vi "Teleop.vi"(10 "Match Info":T4={"Autonomous Elapsed Seconds"=0.0, "TeleOp Elapsed Seconds"=0.0, "Disabled Elapsed Seconds"=0.0, "Visited Autonomous"=FALSE, "Visited TeleOp"=FALSE, "Visited Disabled"=FALSE, "Autonomous Settings"={"Autonomous Style"=enum."Independent", "VI Refnum"=refnum}}, 11 "Call Context":T5) -> ()   [LabVIEW 2013]
doc: "This VI is called for each TeleOp packet received from the DS where the robot is not disabled. It is often used to read from the joysticks and update I/O or to update setpoints for timed control loops. It should complete and return within 20 milliseconds or it may miss DS packets."
uses:
  <vilib>/Rock Robotics/WPI/DriverStation/WPI_DriverStationDerivedRobotMode.ctl
  <vilib>/Rock Robotics/WPI/DriverStation/WPI_DriverStationMatch Info.ctl
  <vilib>/Rock Robotics/WPI/Solenoid/WPI_SolenoidValue.ctl
  <vilib>/Rock Robotics/WPI/Relay/WPI_RelayValue.ctl
  Robot Global Data.vi
  <vilib>/Rock Robotics/Network Tables/SD Read Number.vi
  <vilib>/Rock Robotics/WPI/Solenoid/WPI_SolenoidGetEnum.vi
  <vilib>/Rock Robotics/WPI/Solenoid/WPI_SolenoidSetEnum.vi
  <vilib>/Rock Robotics/WPI/Compressor/WPI_CompressorGetSetRefNum.vi
  <vilib>/Rock Robotics/WPI/Joystick/WPI_JoystickGetSetRefNum.vi
  <vilib>/Rock Robotics/WPI/RobotDrive/WPI_RobotDriveGetSetRefNum.vi
panel:
  out "Waveform Chart 4":dbl(graph)
  out "Waveform Chart 3":dbl(graph)
  in  "Grabber Timer":dbl
  in  "GrabberCurrentTarget":dbl
  in  "HasGrabberBeenReset":bool
  in  "ToughBoxEncoderTopPosition":dbl
  in  "Current Grabber Status":T1(ring)
  out "Waveform Chart 2":dbl(graph)
  in  "Run Grabber PID 2":bool
  out "Reed Switch 2":bool
  out "Reed Switch 1":bool
  out "Top Limit Tripped":bool
  out "Micro Switch":bool
  out "Bottom Limit Tripped":bool
  out "Axis Value  6":dbl
  out "Axis Value 5":dbl
  out "Axis Value 4":dbl
  in  "Grabber Axis Value":T2(ring)
  in  "Current Shooter Status":T3(ring)
  out "Waveform Chart":dbl(graph)
  out "Mechanism Moving Up":bool
  out "Mechanism Moving Down":bool
  out "Time Since Button Pressed":dbl
  in  "Manual Override Activated":bool
  in  "Button 2 Pressed":bool
  in  "Firing Pin Forward":bool
  in  "Mechanism Piston Forward":bool
  in  "Tick Taken":bool
  out "Time at Gather":dbl
  out "Timer for firing mech":dbl
  in  "Mechanism Status":string
types:
  T1 = enum16{"Resetting", "Going Up", "Going Up Slow", "In Shooting Position", "Going Down", "Going Down Slow", "In Loading Position"}
  T2 = enum16{"Less Than Zero", "Greater Than Zero", "Equal To Zero"}
  T3 = enum16{"Retracting", "Firing", "Ready to fire", "Pulling back", "Just fired"}
  T4 = typedef "WPI_DriverStationMatch Info.ctl" = cluster{"Autonomous Elapsed Seconds":dbl, "TeleOp Elapsed Seconds":dbl, "Disabled Elapsed Seconds":dbl, "Visited Autonomous":bool, "Visited TeleOp":bool, "Visited Disabled":bool, "Autonomous Settings":cluster{"Autonomous Style":enum16{"Iterative", "Independent"}, "VI Refnum":refnum<vi>}}
  T5 = typedef "WPI_DriverStationDerivedRobotMode.ctl" = enum16{"Init", "Execute", "Stop"}
  T6 = typedef "WPI_SolenoidValue.ctl" = enum16{"Off", "On", "Forward", "Reverse"}
  T7 = enum16{"Resetting", "Going Up", "Going Up Slow", "In Shooting Position", "Going Down", "Going Down Slow", "In Loading Position", ""}
  T8 = typedef "WPI_MotorControlDeviceRef.ctl" = cluster{"DeviceStatus":errorcluster, "Type":enum16{"PWM", "CAN"}, "PWM":cluster{"Digital Module":T9, "PWM Channel":T10, "DeadBand":T11}, "CAN":cluster{"Device Number":u8, "Control Mode":T12, "Semaphore":T13, "Max Vout":dbl}, "Invert":bool, "TransformRef":T14, "InvTransformRef":T14}
  T9 = typedef "FPGA_TypedefDigitalModule.ctl" = enum16{"Digital Module 1", "Digital Module 2"}
  T10 = typedef "FPGA_DIOPWMChannel.ctl" = enum8{"PWM 1", "PWM 2", "PWM 3", "PWM 4", "PWM 5", "PWM 6", "PWM 7", "PWM 8", "PWM 9", "PWM 10", "Invalid"}
  T11 = typedef "WPI_PWMDeadband.ctl" = cluster{"Name":string, "maxPositivePwm":i32, "minPositivePwm":i32, "centerPwm":i32, "maxNegativePwm":i32, "minNegativePwm":i32, "angularRange":u16}
  T12 = typedef "WPI_CANJaguar_ControlMode.ctl" = enum8{"Percent VBus", "Current", "Speed", "Position", "Voltage"}
  T13 = typedef "Semaphore RefNum" = refnum<k1>
  T14 = typedef "WPI_PWMTransform_ConPane.ctl" = refnum<vi>
  T15 = typedef "WPI_SolenoidDevRef.ctl" = cluster{"DevStatus":errorcluster, "Solenoid Module":T16, "Forward Solenoid Channel":T17, "Reverse Solenoid Channel":T17}
  T16 = typedef "FPGA_TypedefSolenoidModule.ctl" = enum16{"Solenoid Module 1", "Solenoid Module 2"}
  T17 = typedef "WPI_SolenoidChannel.ctl" = enum8{"Solenoid 1", "Solenoid 2", "Solenoid 3", "Solenoid 4", "Solenoid 5", "Solenoid 6", "Solenoid 7", "Solenoid 8", "Invalid"}
  T18 = typedef "WPI_JoystickDevRef.ctl" = cluster{"Device":T19}
  T19 = typedef "WPI_JoystickDeviceEnum.ctl" = enum16{"USB 1", "USB 2", "USB 3", "USB 4", "Kinect 1", "Kinect 2"}
  T20 = typedef "WPI_JoystickButtonState.ctl" = cluster{"Button 1":bool, "Button 2":bool, "Button 3":bool, "Button 4":bool, "Button 5":bool, "Button 6":bool, "Button 7":bool, "Button 8":bool, "Button 9":bool, "Button 10":bool, "Button 11":bool, "Button 12":bool}
  T21 = typedef "WPI_DigitalInputDevRef.ctl" = cluster{"DevStatus":errorcluster, "DIO Channel":T22, "Digital Module":T9}
  T22 = typedef "FPGA_DIOChannel.ctl" = enum8{"DIO 1", "DIO 2", "DIO 3", "DIO 4", "DIO 5", "DIO 6", "DIO 7", "DIO 8", "DIO 9", "DIO 10", "DIO 11", "DIO 12", "DIO 13", "DIO 14", "Invalid"}
  T23 = typedef "WPI_EncoderDevRef.ctl" = cluster{"DevStatus":errorcluster, "EncoderIndex":T24, "CounterIndex":T25, "DistancePerCount":dbl, "Decoding Type":T26}
  T24 = typedef "FPGA_EncoderIdx.ctl" = enum8{"Enc 0", "Enc 1", "Enc 2", "Enc 3", "Invalid"}
  T25 = typedef "FPGA_CounterCtrSystemIndex.ctl" = enum8{"Ctr 0", "Ctr 1", "Ctr 2", "Ctr 3", "Ctr 4", "Ctr 5", "Ctr 6", "Ctr 7", "Invalid"}
  T26 = typedef "WPI_EncoderType.ctl" = enum16{"1x", "2x", "4x"}
  T27 = typedef "WPI_RelayDevRef.ctl" = cluster{"DevStatus":errorcluster, "Relay Channel":T28, "Digital Module":T9, "Relay Direction":T29}
  T28 = typedef "FPGA_DIORelayChannel.ctl" = enum8{"Relay 1", "Relay 2", "Relay 3", "Relay 4", "Relay 5", "Relay 6", "Relay 7", "Relay 8", "Invalid"}
  T29 = typedef "WPI_RelayDirection.ctl" = enum16{"Both directions", "Forward only", "Reverse only"}
  T30 = typedef "WPI_CompressorDevRef.ctl" = cluster{"DevStatus":errorcluster, "DigitalInputDevRef":T21, "RelayDevRef":T27}
  T31 = typedef "WPI_RelayValue.ctl" = enum16{"Off", "On", "Forward", "Reverse"}
  T32 = typedef "WPI_AnalogChannelDevRef.ctl" = cluster{"DevStatus":errorcluster, "Analog Module":T33, "Analog Channel":T34}
  T33 = typedef "FPGA_TypedefAnalogModule.ctl" = enum16{"Analog Module 1", "Analog Module 2"}
  T34 = typedef "FPGA_AIChannel.ctl" = enum8{"AI 1", "AI 2", "AI 3", "AI 4", "AI 5", "AI 6", "AI 7", "AI 8", "Invalid"}
  T35 = typedef "WPI_ServoDeviceRef.ctl" = cluster{"DeviceStatus":errorcluster, "Digital Module":T9, "PWM Channel":T10, "DeadBand":T11}
  T36 = cluster{"axis 1 (x)":dbl, "axis 2 (y)":dbl, "axis 3 (throttle)":dbl, "axis 4":dbl, "axis 5":dbl, "axis 6":dbl}
  T37 = typedef "WPI_RobotDriveDevRef.ctl" = cluster{"DevStatus":errorcluster, "Motors[]":T8[], "Square Inputs":bool, "Max Output":dbl, "Isochronous":bool}
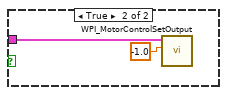
[diagram p2: hidden frame]
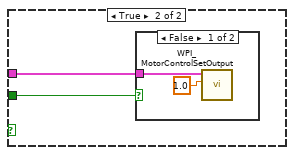
[diagram p3: hidden frame]
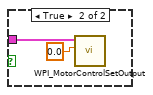
[diagram p4: hidden frame]
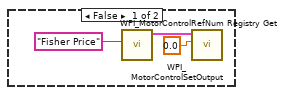
[diagram p5: hidden frame]
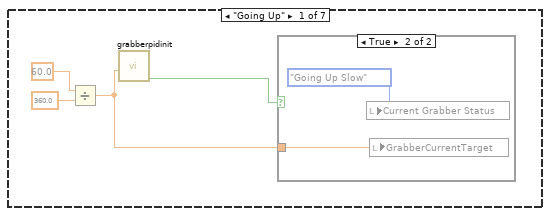
[diagram p7: hidden frame]
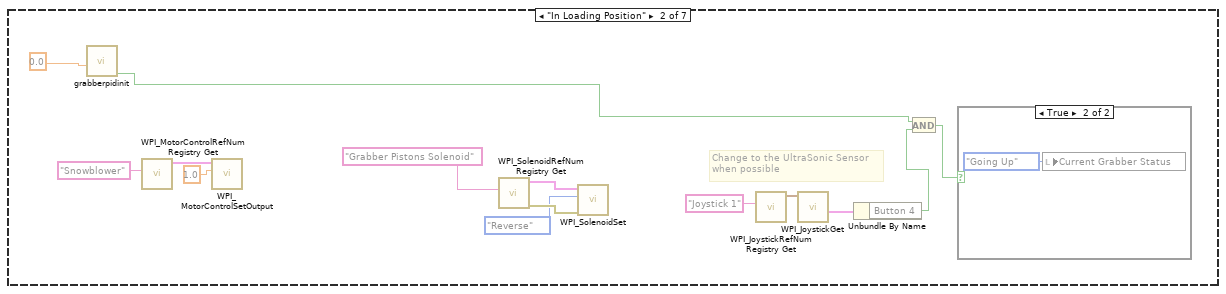
[diagram p9: hidden frame]
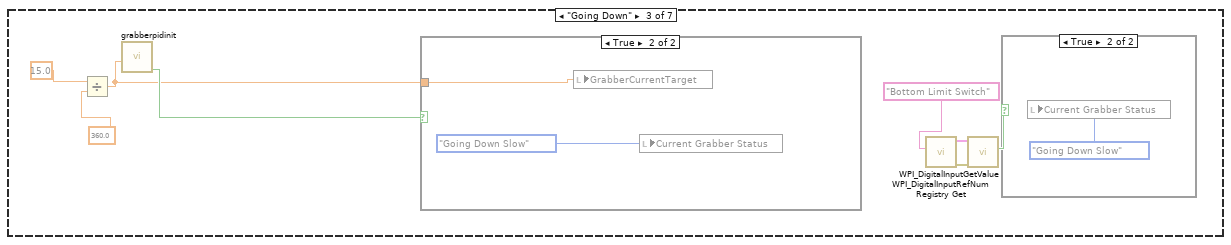
[diagram p11: hidden frame]
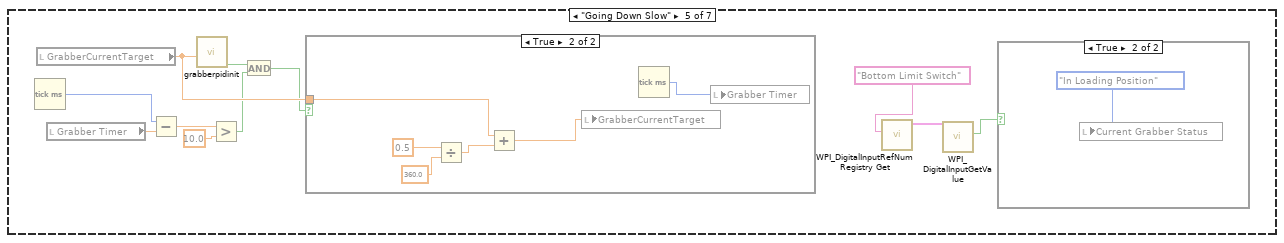
[diagram p15: hidden frame]
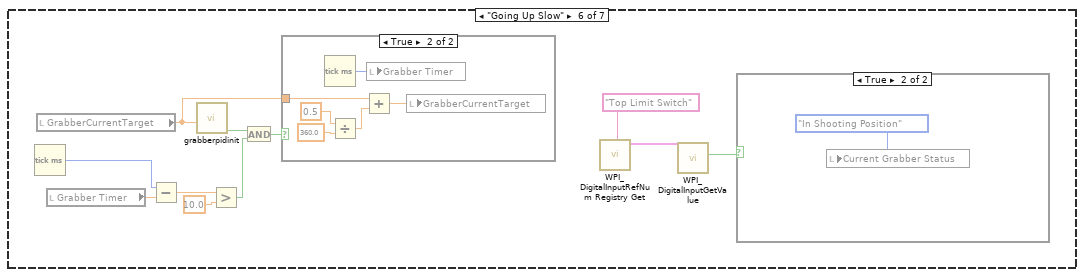
[diagram p18: hidden frame]
diagram:
  (unwired) "Below code is for running the Raising/Lowering motors"
  (unwired) "This code sets the toggle rate used by the Periodic Tasks VI.  For teleop mode we flash the USER1 LED on the cRIO at a fast rate.  Look at the Periodic Tasks VI to see how this global value is used."
  (unwired) "This VI is called each time a TeleOp DS packet is received.  Use it to respond to new joystick or Driver Station values.\n\nCommon tasks include reading the joysticks and updating motors, and updating setpoints for periodic loops.\n\nYou can open I/O on the FIRST Call, or in the Begin.vi."
  # "Top Limit Switch may need invert"
  # "one encoder"
  # "Check me!"
  # "If no buttons pressed - 0\nIf left pressed = 7\nIf right pressed = -7\nIf both = 0"
  # "Publish the Robot Drive Motor\nvalues to the dashboard"
  # "Publish the joystick data the\nrobot sees to the dashboard"
  # "Each time we enter, report that\nwe are running teleop"
  # "Use to differentiate between\nFirst, Last, and Intermediate calls"
  # "Read Joystick X and Y values and update motor values"
  n1 = call <vilib>:"SD Read Boolean.vi"("Name"="Manual Mechanism Override") -> ("Boolean"=w54:bool)  [unwired: 8 in, 2 out]
  n2 = disable-structure shown="Disabled" {
    disable-tunnel: w54 -> [w153 _]
    frame Disabled {
      n3 = Not(x=w153) -> (.not. x?=w154:bool)
      n4 = case shown="True" w154 {
        frame False {
        }
        frame True {
          n5 = local read "Current Grabber Status"() -> (w155:T1)
          n6 = case shown="\"In Shooting Position\"" w155 {
            frame "Going Up" {
              n7 = Divide(x=60.0 ("setpoint"), y=360.0) -> (x/y=w158:dbl)
              n8 = call "grabberpidinit.vi"("setpoint"=w158) -> ("Done? 2"=w159:bool)  [unwired: 10 in]
              n9 = case shown="True" w159 {
                tunnel: w158 -> [_ w160]
                frame False {
                }
                frame True {
                  n10 = local write "Current Grabber Status"(T1."Going Up Slow" ("Current Grabber Status")) -> ()
                  n11 = local write "GrabberCurrentTarget"(w160) -> ()
                }
              }
            }
            frame "In Loading Position" {
              # "Change to the UltraSonic Sensor\nwhen possible"
              n12 = call "grabberpidinit.vi"("setpoint"=0.0) -> ("Done? 2"=w162:bool)  [unwired: 10 in]
              n13 = call <vilib>:"WPI_MotorControlRefNum Registry Get.vi"("refnum name"="Snowblower") -> ("MotorControlDevRef"=w174:T8)  [unwired: 9 in, 1 out]
              n14 = call <vilib>:"WPI_MotorControlSetOutput.vi"("Output"=1.0, "MotorControlDevRef"=w174) -> ()  [unwired: 7 in, 3 out]
              n15 = call <vilib>:"WPI_SolenoidRefNum Registry Get.vi"("refnum name"="Grabber Pistons Solenoid") -> ("error out"=w171:errorcluster, "SolenoidDevRef"=w170:T15)  [unwired: 9 in]
              n16 = call-poly <vilib>:"WPI_SolenoidSet.vi"("error in (no error)"=w171, "Value"=WPI_SolenoidValue."Reverse", "SolenoidDevRef"=w170) -> ()  [unwired: 7 in, 2 out]
              n17 = call <vilib>:"WPI_JoystickRefNum Registry Get.vi"("refnum name"="Joystick 1") -> ("JoystickDevRef"=w166:T18)  [unwired: 1 in, 9 out]
              n18 = call <vilib>:"WPI_JoystickGet.vi"("JoystickDevRef"=w166) -> ("Buttons"=w165:T20)  [unwired: 1 in, 5 out]
              n19 = Unbundle By Name(w165) -> ("Button 4"=w163:bool)
              n20 = And(x=w162, y=w163) -> (x .and. y?=w164:bool)
              n21 = case shown="True" w164 {
                frame False {
                }
                frame True {
                  n22 = local write "Current Grabber Status"(T1."Going Up" ("Current Grabber Status")) -> ()
                }
              }
            }
            frame "Going Down" {
              n23 = Divide(x=15.0, y=360.0) -> (x/y=w181:dbl)
              n24 = call "grabberpidinit.vi"("setpoint"=w181) -> ("Done? 2"=w182:bool)  [unwired: 10 in]
              n25 = case shown="True" w182 {
                tunnel: w181 -> [_ w187]
                frame False {
                }
                frame True {
                  n26 = local write "GrabberCurrentTarget"(w187) -> ()
                  n27 = local write "Current Grabber Status"(T1."Going Down Slow" ("Current Grabber Status")) -> ()
                }
              }
              n28 = call <vilib>:"WPI_DigitalInputRefNum Registry Get.vi"("refnum name"="Bottom Limit Switch") -> ("error out"=w179:errorcluster, "DigitalInputDevRef"=w178:T21)  [unwired: 9 in]
              n29 = call <vilib>:"WPI_DigitalInputGetValue.vi"("error in (no error)"=w179, "DigitalInputDevRef"=w178) -> ("Value"=w177:bool)  [unwired: 7 in, 2 out]
              n30 = case shown="True" w177 {
                frame False {
                }
                frame True {
                  n31 = local write "Current Grabber Status"(T1."Going Down Slow" ("Current Grabber Status")) -> ()
                }
              }
            }
            frame "In Shooting Position" {
              n32 = local read "ToughBoxEncoderTopPosition"() -> (w189:dbl)
              n33 = call <vilib>:"WPI_JoystickRefNum Registry Get.vi"("refnum name"="Joystick 1") -> ("JoystickDevRef"=w191:T18)  [unwired: 1 in, 9 out]
              n34 = call <vilib>:"WPI_JoystickGet.vi"("JoystickDevRef"=w191) -> ("Buttons"=w190:T20)  [unwired: 1 in, 5 out]
              n35 = Unbundle By Name(w190) -> ("Button 1"=w188:bool)
              n36 = case shown="True" w188 {
                frame False {
                }
                frame True {
                  n37 = local write "Current Grabber Status"(T7."Going Down" ("Current Grabber Status")) -> ()
                }
              }
              n38 = call "grabberpidinit.vi"("setpoint"=w189, "reinitialize? (F) 2"=w188) -> ()  [unwired: 9 in, 1 out]
            }
            frame "Going Down Slow" {
              n39 = Tick Count (ms)() -> (millisecond timer value=w203:u32)
              n40 = local read "GrabberCurrentTarget"() -> (w204:dbl)
              n41 = local read "Grabber Timer"() -> (w200:dbl)
              n42 = Subtract(x=w203, y=w200) -> (x-y=w202:dbl)
              n43 = call "grabberpidinit.vi"("setpoint"=w204) -> ("Done? 2"=w198:bool)  [unwired: 10 in]
              n44 = Greater?(x=w202, y=10.0) -> (0:w199:bool)
              n45 = And(x=w198, y=w199) -> (x .and. y?=w197:bool)
              n46 = case shown="True" w197 {
                tunnel: w204 -> [_ w208]
                frame False {
                }
                frame True {
                  n47 = Divide(x=0.5, y=360.0) -> (x/y=w209:dbl)
                  n48 = Add(x=w208, y=w209) -> (x+y=w207:dbl)
                  n49 = local write "GrabberCurrentTarget"(w207) -> ()
                  n50 = Tick Count (ms)() -> (millisecond timer value=w206:u32)
                  n51 = local write "Grabber Timer"(w206) -> ()
                }
              }
              n52 = call <vilib>:"WPI_DigitalInputRefNum Registry Get.vi"("refnum name"="Bottom Limit Switch") -> ("DigitalInputDevRef"=w195:T21)  [unwired: 9 in, 1 out]
              n53 = call <vilib>:"WPI_DigitalInputGetValue.vi"("DigitalInputDevRef"=w195) -> ("Value"=w194:bool)  [unwired: 8 in, 2 out]
              n54 = case shown="True" w194 {
                frame False {
                }
                frame True {
                  n55 = local write "Current Grabber Status"(T1."In Loading Position" ("Current Grabber Status")) -> ()
                }
              }
            }
            frame "Going Up Slow" {
              n56 = Tick Count (ms)() -> (millisecond timer value=w221:u32)
              n57 = local read "GrabberCurrentTarget"() -> (w222:dbl)
              n58 = local read "Grabber Timer"() -> (w220:dbl)
              n59 = Subtract(x=w221, y=w220) -> (x-y=w219:dbl)
              n60 = call "grabberpidinit.vi"("setpoint"=w222) -> ("Done? 2"=w217:bool)  [unwired: 10 in]
              n61 = Greater?(x=w219, y=10.0) -> (0:w216:bool)
              n62 = And(x=w217, y=w216) -> (x .and. y?=w215:bool)
              n63 = case shown="True" w215 {
                tunnel: w222 -> [_ w228]
                frame False {
                }
                frame True {
                  n64 = Tick Count (ms)() -> (millisecond timer value=w224:u32)
                  n65 = Divide(x=0.5 ("y"), y=360.0) -> (x/y=w225:dbl)
                  n66 = Add(x=w228, y=w225) -> (x+y=w229:dbl)
                  n67 = local write "Grabber Timer"(w224) -> ()
                  n68 = local write "GrabberCurrentTarget"(w229) -> ()
                }
              }
              n69 = call <vilib>:"WPI_DigitalInputRefNum Registry Get.vi"("refnum name"="Top Limit Switch") -> ("DigitalInputDevRef"=w213:T21)  [unwired: 9 in, 1 out]
              n70 = call <vilib>:"WPI_DigitalInputGetValue.vi"("DigitalInputDevRef"=w213) -> ("Value"=w212:bool)  [unwired: 8 in, 2 out]
              n71 = case shown="True" w212 {
                frame False {
                }
                frame True {
                  n72 = local write "Current Grabber Status"(T1."In Shooting Position" ("Current Grabber Status")) -> ()
                }
              }
            }
            frame "Resetting", Default {
              n73 = local read "GrabberCurrentTarget"() -> (w243:dbl)
              n74 = call <vilib>:"WPI_DigitalInputRefNum Registry Get.vi"("refnum name"="Bottom Limit Switch") -> ("DigitalInputDevRef"=w233:T21)  [unwired: 9 in, 1 out]
              n75 = call <vilib>:"WPI_DigitalInputGetValue.vi"("DigitalInputDevRef"=w233) -> ("Value"=w231:bool)  [unwired: 8 in, 2 out]
              n76 = Equal?(x=w243, y=0.0) -> (x = y?=w242:bool)
              n77 = Not(x=w231) -> (.not. x?=w230:bool)
              n78 = case shown="True" w242 {
                tunnel: [w255 w256] -> w241
                tunnel: w243 -> [w255 _]
                frame False {
                }
                frame True {
                  # "one encoder"
                  n79 = call <vilib>:"WPI_EncoderRefNum Registry Get.vi"("refnum name"="Tough Box Encoder") -> ("error out"=w267:errorcluster, "EncoderDevRef"=w266:T23)  [unwired: 9 in]
                  n80 = call <vilib>:"WPI_EncoderGet.vi"("error in (no error)"=w267, "EncoderDevRef"=w266) -> ("Distance"=w259:dbl)  [unwired: 4 in, 5 out]
                  n81 = Divide(x=w259, y=360.0) -> (x/y=w262:dbl)
                  n82 = Multiply(x=w262, y=12.0) -> (x*y=w263:dbl)
                  n83 = Divide(x=w263, y=60.0) -> (x/y=w258:dbl)
                  n84 = Multiply(x=w258, y=1.5) -> (x*y=w256:dbl)
                  n85 = local write "GrabberCurrentTarget"(w256) -> ()
                }
              }
              n86 = case shown="True" w230 {
                frame False {
                }
                frame True {
                  n87 = local write "Current Grabber Status"(T7."In Loading Position" ("Current Grabber Status")) -> ()
                  n88 = call <vilib>:"WPI_EncoderRefNum Registry Get.vi"("refnum name"="Tough Box Encoder") -> ("error out"=w247:errorcluster, "EncoderDevRef"=w246:T23)  [unwired: 9 in]
                  n89 = call <vilib>:"WPI_EncoderReset.vi"("error in (no error)"=w247, "EncoderDevRef"=w246) -> ()  [unwired: 8 in, 2 out]
                }
              }
              n90 = local read "Grabber Timer"() -> (w239:dbl)
              n91 = Tick Count (ms)() -> (millisecond timer value=w240:u32)
              n92 = Subtract(x=w240, y=w239) -> (x-y=w238:dbl)
              n93 = call "grabberpidinit.vi"("setpoint"=w241, "reinitialize? (F) 2"=w230) -> ("Done? 2"=w234:bool)  [unwired: 9 in]
              n94 = Greater?(x=w238, y=10.0) -> (0:w235:bool)
              n95 = And(x=w234, y=w235) -> (x .and. y?=w236:bool)
              n96 = case shown="True" w236 {
                tunnel: w241 -> [_ w251]
                frame False {
                }
                frame True {
                  n97 = Tick Count (ms)() -> (millisecond timer value=w249:u32)
                  n98 = Divide(x=0.5, y=360.0) -> (x/y=w254:dbl)
                  n99 = Subtract(x=w251, y=w254) -> (x-y=w250:dbl)
                  n100 = local write "Grabber Timer"(w249) -> ()
                  n101 = local write "GrabberCurrentTarget"(w250) -> ()
                }
              }
            }
          }
        }
      }
    }
    frame Enabled {
    }
  }
  n102 = local write "Mechanism Piston Forward"(FALSE) -> ()
  n103 = local write "Firing Pin Forward"(FALSE) -> ()
  n104 = call <vilib>:"WPI_DriverStationReport Robot Code State.vi"("TeleOp"=TRUE ("Autonomous")) -> ()  [unwired: 10 in, 1 out]
  n105 = global write "Robot Global Data.vi" "LED toggle rate (ms)"(u32 100 ("LED ms toggle rate")) -> ()
  n106 = call <vilib>:"WPI_JoystickRefNum Registry Get.vi"("refnum name"="Joystick 1") -> ("JoystickDevRef"=w131:T18)  [unwired: 1 in, 9 out]
  n107 = Unbundle By Name("Match Info") -> ()  [unwired: 1 out]
  n108 = call <vilib>:"SD Read Boolean.vi"("Name"="Light Ring On") -> ("Boolean"=w62:bool)  [unwired: 8 in, 2 out]
  n109 = call <vilib>:"WPI_RelayRefNum Registry Get.vi"("refnum name"="Light Ring") -> ("RelayDevRef"=w61:T27)  [unwired: 9 in, 1 out]
  n110 = call <vilib>:"WPI_DigitalInputRefNum Registry Get.vi"("refnum name"="Reed Switch 1") -> ("DigitalInputDevRef"=w80:T21)  [unwired: 9 in, 1 out]
  n111 = call <vilib>:"WPI_DigitalInputRefNum Registry Get.vi"("refnum name"="Reed Switch 2") -> ("DigitalInputDevRef"=w73:T21)  [unwired: 9 in, 1 out]
  n112 = call <vilib>:"WPI_DigitalInputRefNum Registry Get.vi"("refnum name"="Reed Switch 2") -> ("DigitalInputDevRef"=w77:T21)  [unwired: 9 in, 1 out]
  n113 = call <vilib>:"WPI_DigitalInputRefNum Registry Get.vi"("refnum name"="Micro Switch 1") -> ("DigitalInputDevRef"=w92:T21)  [unwired: 9 in, 1 out]
  n114 = call <vilib>:"WPI_DigitalInputRefNum Registry Get.vi"("refnum name"="Micro Switch 1") -> ("DigitalInputDevRef"=w69:T21)  [unwired: 9 in, 1 out]
  n115 = call <vilib>:"WPI_DigitalInputRefNum Registry Get.vi"("refnum name"="Top Limit Switch") -> ("DigitalInputDevRef"=w85:T21)  [unwired: 9 in, 1 out]
  n116 = call <vilib>:"WPI_JoystickGet.vi"("JoystickDevRef"=w131) -> ("Buttons"=w130:T20)  [unwired: 1 in, 5 out]
  n117 = call <vilib>:"SD Read Boolean.vi"("Name"="Compressor On/Off") -> ("Boolean"=w94:bool)  [unwired: 8 in, 2 out]
  n118 = call <vilib>:"WPI_CompressorRefNum Registry Get.vi"("refnum name"="Compressor") -> ("CompressorDevRef"=w95:T30)  [unwired: 9 in, 1 out]
  n119 = call <vilib>:"WPI_DigitalInputRefNum Registry Get.vi"("refnum name"="Bottom Limit Switch") -> ("DigitalInputDevRef"=w100:T21)  [unwired: 9 in, 1 out]
  n120 = case shown="False" w62 {
    tunnel: w61 -> [w268 w271]
    frame False {
      n121 = call <vilib>:"WPI_RelaySet.vi"("RelayValue"=WPI_RelayValue."Off", "RelayDevRef"=w268) -> ()  [unwired: 8 in, 2 out]
    }
    frame True {
      n122 = call <vilib>:"WPI_RelaySet.vi"("RelayValue"=WPI_RelayValue."Forward", "RelayDevRef"=w271) -> ()  [unwired: 8 in, 2 out]
    }
  }
  n123 = call <vilib>:"WPI_DigitalInputGetValue.vi"("DigitalInputDevRef"=w80) -> ("Value"=→"Reed Switch 1":bool)  [unwired: 8 in, 2 out]
  n124 = call <vilib>:"WPI_DigitalInputGetValue.vi"("DigitalInputDevRef"=w73) -> ("Value"=w72:bool)  [unwired: 8 in, 2 out]
  n125 = call <vilib>:"WPI_DigitalInputGetValue.vi"("DigitalInputDevRef"=w77) -> ("Value"=→"Reed Switch 2":bool)  [unwired: 8 in, 2 out]
  n126 = call <vilib>:"WPI_DigitalInputGetValue.vi"("DigitalInputDevRef"=w92) -> ("Value"=→"Micro Switch":bool)  [unwired: 8 in, 2 out]
  n127 = call <vilib>:"WPI_DigitalInputGetValue.vi"("DigitalInputDevRef"=w69) -> ("Value"=w68:bool)  [unwired: 8 in, 2 out]
  n128 = call <vilib>:"WPI_DigitalInputGetValue.vi"("DigitalInputDevRef"=w85) -> ("Value"=→"Top Limit Tripped":bool)  [unwired: 8 in, 2 out]
  n129 = Unbundle By Name(w130) -> ("Button 8"=w129:bool)
  n130 = call <vilib>:"WPI_AnalogChannelRefNum Registry Get.vi"("refnum name"="Grabber Ultrasonic Sensor") -> ("AIDeviceRef"=w59:T32)  [unwired: 9 in, 1 out]
  n131 = case shown="False" w94 {
    tunnel: w95 -> [w272 w273]
    frame False {
      n132 = call <vilib>:"WPI_CompressorStop.vi"("CompressorDevRef"=w272) -> ()  [unwired: 9 in, 2 out]
    }
    frame True {
      n133 = call <vilib>:"WPI_CompressorStart.vi"("CompressorDevRef"=w273) -> ()  [unwired: 9 in, 2 out]
    }
  }
  n134 = call <vilib>:"WPI_DigitalInputGetValue.vi"("DigitalInputDevRef"=w100) -> ("Value"=→"Bottom Limit Tripped":bool)  [unwired: 8 in, 2 out]
  n135 = Not(x=w72) -> (.not. x?=w71:bool)
  n136 = call-poly <vilib>:"SD Read Value.vi"("Name"="Camera Pitch Control") -> ("Numeric"=w113:dbl)  [unwired: 8 in, 2 out]
  n137 = call <vilib>:"WPI_SolenoidRefNum Registry Get.vi"("refnum name"="Grabber Pistons Solenoid") -> ("SolenoidDevRef"=w9:T15)  [unwired: 9 in, 1 out]
  n138 = call <vilib>:"SD Read Boolean.vi"("Name"="Manual Mechanism Override") -> ("Boolean"=w81:bool)  [unwired: 8 in, 2 out]
  n139 = call <vilib>:"WPI_SolenoidRefNum Registry Get.vi"("refnum name"="Drawback Pistons") -> ("SolenoidDevRef"=w122:T15)  [unwired: 9 in, 1 out]
  n140 = call <vilib>:"WPI_SolenoidRefNum Registry Get.vi"("refnum name"="Firing Pin Solenoid") -> ("SolenoidDevRef"=w124:T15)  [unwired: 9 in, 1 out]
  n141 = Not(x=w68) -> (.not. x?=w67:bool)
  n142 = call <vilib>:"WPI_ServoRefNum Registry Get.vi"("refnum name"="Camera Pitch Servo") -> ("ServoDeviceRef"=w114:T35)  [unwired: 9 in, 1 out]
  n143 = call-poly <vilib>:"SD Read Value.vi"("Name"="Camera Rotation Control") -> ("Numeric"=w117:dbl)  [unwired: 8 in, 2 out]
  n144 = call <vilib>:"WPI_AnalogChannelGetVoltage.vi"("AIDeviceRef"=w59) -> ("Voltage"=→"Waveform Chart":dbl)  [unwired: 8 in, 2 out]
  n145 = call <vilib>:"WPI_ServoRefNum Registry Get.vi"("refnum name"="Camera Rotation Servo") -> ("ServoDeviceRef"=w116:T35)  [unwired: 9 in, 1 out]
  n146 = call <vilib>:"SD Write Boolean.vi"("Boolean"=w71, "Name"="Are Drawback Pistons Extended") -> ()  [unwired: 8 in, 2 out]
  n147 = call <vilib>:"SD Write Boolean.vi"("Boolean"=w67, "Name"="Is The Firing Pin Piston Extended") -> ()  [unwired: 8 in, 2 out]
  n148 = call <vilib>:"SD Read Boolean.vi"("Name"="Manual Mechanism Override") -> ("Boolean"=w107:bool)  [unwired: 8 in, 2 out]
  n149 = call-poly <vilib>:"WPI_SolenoidGet.vi"("SolenoidDevRef"=w9) -> ("Value"=w104:T6)  [unwired: 8 in, 2 out]
  n150 = call <vilib>:"WPI_JoystickRefNum Registry Get.vi"("refnum name"="Joystick 1") -> ("JoystickDevRef"=w136:T18)  [unwired: 1 in, 9 out]
  n151 = call <vilib>:"WPI_DigitalInputRefNum Registry Get.vi"("refnum name"="Bottom Limit Switch") -> ("DigitalInputDevRef"=w41:T21)  [unwired: 9 in, 1 out]
  n152 = call <vilib>:"WPI_ServoSetAngle.vi"("Angle"=w113, "ServoDeviceRef"=w114) -> ()  [unwired: 8 in, 2 out]
  n153 = case shown="True" w81 {
    tunnel: w124 -> [_ w284]
    tunnel: w122 -> [_ w283]
    frame False {
    }
    frame True {
      n154 = call <vilib>:"SD Read Boolean.vi"("Name"="Drawback Pistons Activated") -> ("Boolean"=w274:bool)  [unwired: 8 in, 2 out]
      n155 = call <vilib>:"SD Read Boolean.vi"("Name"="Firing Pin Piston Extended") -> ("Boolean"=w281:bool)  [unwired: 8 in, 2 out]
      n156 = case shown="True" w274 {
        tunnel: w283 -> [_ w292]
        frame False {
        }
        frame True {
          n157 = call <vilib>:"SD Read Boolean.vi"("Name"="Drawback Piston Extended") -> ("Boolean"=w290:bool)  [unwired: 8 in, 2 out]
          n158 = Equal?(x=w290, y=FALSE) -> (x = y?=w288:bool)
          n159 = Select(t=WPI_SolenoidValue."Forward" ("Value"), s=w288, f=WPI_SolenoidValue."Reverse") -> (s? t:f=w285:T6)
          n160 = call-poly <vilib>:"WPI_SolenoidSet.vi"("Value"=w285, "SolenoidDevRef"=w292) -> ()  [unwired: 8 in, 2 out]
        }
      }
      n161 = Equal?(x=w281, y=FALSE) -> (x = y?=w277:bool)
      n162 = Select(t=WPI_SolenoidValue."Forward" ("Value"), s=w277, f=WPI_SolenoidValue."Reverse") -> (s? t:f=w278:T6)
      n163 = call-poly <vilib>:"WPI_SolenoidSet.vi"("Value"=w278, "SolenoidDevRef"=w284) -> ()  [unwired: 8 in, 2 out]
    }
  }
  n164 = call <vilib>:"WPI_ServoSetAngle.vi"("Angle"=w117, "ServoDeviceRef"=w116) -> ()  [unwired: 8 in, 2 out]
  n165 = Equal?(x=w104, y=WPI_SolenoidValue."Forward") -> (x = y?=w57:bool)
  n166 = case shown="True" w129 {
    frame False {
    }
    frame True {
      n167 = global read "Robot Global Data.vi" "Time since  button 8 pressed"() -> (w293:dbl)
      n168 = Tick Count (ms)() -> (millisecond timer value=w297:u32)
      n169 = Subtract(x=w297, y=w293) -> (x-y=w296:dbl)
      n170 = Greater?(x=w296, y=300) -> (0:w294:bool)
      n171 = case shown="True" w294 {
        frame False {
        }
        frame True {
          n172 = Tick Count (ms)() -> (millisecond timer value=w298:u32)
          n173 = local read "Manual Override Activated"() -> (w302:bool)
          n174 = global write "Robot Global Data.vi" "Time since  button 8 pressed"(w298) -> ()
          n175 = Select(t=FALSE, s=w302, f=TRUE) -> (s? t:f=w299:bool)
          n176 = local write "Manual Override Activated"(w299) -> ()
        }
      }
    }
  }
  n177 = call <vilib>:"WPI_DigitalInputGetValue.vi"("DigitalInputDevRef"=w41) -> ("Value"=w40:bool)  [unwired: 8 in, 2 out]
  n178 = Not(x=w57) -> (.not. x?=w56:bool)
  n179 = call <vilib>:"SD Read Boolean.vi"("Name"="Drawback Pistons Activated") -> ("Boolean"=w89:bool)  [unwired: 8 in, 2 out]
  n180 = Not(x=w107) -> (.not. x?=w88:bool)
  n181 = Not(x=w40) -> (.not. x?=w39:bool)
  n182 = call <vilib>:"WPI_JoystickGet.vi"("JoystickDevRef"=w136) -> ("Buttons"=w135:T20, "Axes"=w128:T36)  [unwired: 1 in, 4 out]
  n183 = call <vilib>:"SD Write Boolean.vi"("Boolean"=w56, "Name"="Are Grabber Pistons Extended") -> ()  [unwired: 8 in, 2 out]
  n184 = case shown="True" w39 {
    frame False {
    }
    frame True {
      n185 = call <vilib>:"WPI_EncoderRefNum Registry Get.vi"("refnum name"="Tough Box Encoder") -> ("error out"=w304:errorcluster, "EncoderDevRef"=w303:T23)  [unwired: 9 in]
      n186 = call <vilib>:"WPI_EncoderReset.vi"("error in (no error)"=w304, "EncoderDevRef"=w303) -> ()  [unwired: 8 in, 2 out]
    }
  }
  n187 = Unbundle By Name(w135) -> ("Button 3"=w43:bool, "Button 5"=w65:bool, "Button 6"=w66:bool)  [unwired: 2 out]
  n188 = And(x=w88, y=w89) -> (x .and. y?=w87:bool)
  n189 = Unbundle By Name(w128) -> ("axis 4"=→"Axis Value 4":dbl, "axis 5"=w83:dbl, "axis 6"=→"Axis Value  6":dbl)
  "Axis Value 5" <- w83
  n190 = Negate(x=w83) -> (-x=w82:dbl)
  n191 = call <vilib>:"WPI_MotorControlRefNum Registry Get.vi"("refnum name"="Snowblower") -> ("MotorControlDevRef"=w17:T8)  [unwired: 9 in, 1 out]
  n192 = local read "Current Grabber Status"() -> (w46:T1)
  n193 = local read "Current Shooter Status"() -> (w47:T3)
  n194 = call <vilib>:"WPI_EncoderRefNum Registry Get.vi"("refnum name"="Tough Box Encoder") -> ("error out"=w50:errorcluster, "EncoderDevRef"=w51:T23)  [unwired: 9 in]
  n195 = case shown="False" w66 {
    tunnel: w65 -> [w307 w313]
    tunnel: w17 -> [w306 w312]
    frame False {
      n196 = case shown="False" w307 {
        tunnel: w306 -> [w309 w311]
        frame False {
          n197 = call <vilib>:"WPI_MotorControlSetOutput.vi"("Output"=0.0, "MotorControlDevRef"=w309) -> ()  [unwired: 7 in, 3 out]
        }
        frame True {
          n198 = call <vilib>:"WPI_MotorControlSetOutput.vi"("Output"=-1.0, "MotorControlDevRef"=w311) -> ()  [unwired: 7 in, 3 out]
        }
      }
    }
    frame True {
      n199 = case shown="False" w313 {
        tunnel: w312 -> [w315 w317]
        frame False {
          n200 = call <vilib>:"WPI_MotorControlSetOutput.vi"("Output"=1.0, "MotorControlDevRef"=w315) -> ()  [unwired: 7 in, 3 out]
        }
        frame True {
          n201 = call <vilib>:"WPI_MotorControlSetOutput.vi"("Output"=0.0, "MotorControlDevRef"=w317) -> ()  [unwired: 7 in, 3 out]
        }
      }
    }
  }
  n202 = case shown="True" w87 {
    tunnel: w43 -> [_ w318]
    frame False {
    }
    frame True {
      n203 = case shown="\"Pulling back\"" "Current Shooter Status" {
        tunnel: w318 -> [_ w326 _ _ _]
        frame "Firing" {
          n204 = Tick Count (ms)() -> (millisecond timer value=w320:u32)
          n205 = local write "Current Shooter Status"(T3."Just fired" ("Current Shooter Status")) -> ()
          n206 = call <vilib>:"WPI_SolenoidRefNum Registry Get.vi"("refnum name"="Firing Pin Solenoid") -> ("error out"=w324:errorcluster, "SolenoidDevRef"=w323:T15)  [unwired: 9 in]
          n207 = call-poly <vilib>:"WPI_SolenoidSet.vi"("error in (no error)"=w324, "Value"=WPI_SolenoidValue."Reverse", "SolenoidDevRef"=w323) -> ()  [unwired: 7 in, 2 out]
          n208 = local write "Timer for firing mech"(w320) -> ()
        }
        frame "Ready to fire" {
          # "Button one is pressed, so fire"
          n209 = case shown="True" w326 {
            frame False {
            }
            frame True {
              n210 = local write "Current Shooter Status"(T3."Firing" ("Current Shooter Status")) -> ()
            }
          }
        }
        frame "Pulling back" {
          # "Need to invert reed switch 2"
          n211 = call <vilib>:"WPI_DigitalInputRefNum Registry Get.vi"("refnum name"="Reed Switch 2") -> ("error out"=w329:errorcluster, "DigitalInputDevRef"=w330:T21)  [unwired: 9 in]
          n212 = call <vilib>:"WPI_DigitalInputGetValue.vi"("error in (no error)"=w329, "DigitalInputDevRef"=w330) -> ("Value"=w328:bool)  [unwired: 7 in, 2 out]
          n213 = call <vilib>:"WPI_SolenoidRefNum Registry Get.vi"("refnum name"="Drawback Pistons") -> ("error out"=w334:errorcluster, "SolenoidDevRef"=w333:T15)  [unwired: 9 in]
          n214 = call <vilib>:"WPI_SolenoidRefNum Registry Get.vi"("refnum name"="Firing Pin Solenoid") -> ("error out"=w338:errorcluster, "SolenoidDevRef"=w337:T15)  [unwired: 9 in]
          n215 = call-poly <vilib>:"WPI_SolenoidSet.vi"("error in (no error)"=w334, "Value"=WPI_SolenoidValue."Forward", "SolenoidDevRef"=w333) -> ()  [unwired: 7 in, 2 out]
          n216 = case shown="True" w328 {
            frame False {
            }
            frame True {
              n217 = Tick Count (ms)() -> (millisecond timer value=w340:u32)
              n218 = local write "Timer for firing mech"(w340) -> ()
              n219 = local write "Current Shooter Status"(T3."Retracting" ("Current Shooter Status")) -> ()
            }
          }
          n220 = call-poly <vilib>:"WPI_SolenoidSet.vi"("error in (no error)"=w338, "Value"=WPI_SolenoidValue."Reverse", "SolenoidDevRef"=w337) -> ()  [unwired: 7 in, 2 out]
        }
        frame "Retracting" {
          n221 = local read "Timer for firing mech"() -> (w355:dbl)
          n222 = call <vilib>:"WPI_DigitalInputRefNum Registry Get.vi"("refnum name"="Reed Switch 1") -> ("error out"=w349:errorcluster, "DigitalInputDevRef"=w350:T21)  [unwired: 9 in]
          n223 = call <vilib>:"WPI_DigitalInputGetValue.vi"("error in (no error)"=w349, "DigitalInputDevRef"=w350) -> ("Value"=w342:bool)  [unwired: 7 in, 2 out]
          n224 = call <vilib>:"WPI_SolenoidRefNum Registry Get.vi"("refnum name"="Firing Pin Solenoid") -> ("error out"=w358:errorcluster, "SolenoidDevRef"=w357:T15)  [unwired: 9 in]
          n225 = Not(x=w342) -> (.not. x?=w343:bool)
          n226 = call-poly <vilib>:"WPI_SolenoidSet.vi"("error in (no error)"=w358, "Value"=WPI_SolenoidValue."Forward", "SolenoidDevRef"=w357) -> ()  [unwired: 7 in, 2 out]
          n227 = Tick Count (ms)() -> (millisecond timer value=w354:u32)
          n228 = case shown="True" w343 {
            frame False {
            }
            frame True {
              n229 = local write "Current Shooter Status"(T3."Ready to fire" ("Current Shooter Status")) -> ()
            }
          }
          n230 = Subtract(x=w354, y=w355) -> (x-y=w345:dbl)
          n231 = Greater Or Equal?(x=w345, y=1000) -> (x >= y?=w347:bool)
          n232 = call <vilib>:"WPI_SolenoidRefNum Registry Get.vi"("refnum name"="Drawback Pistons") -> ("SolenoidDevRef"=w352:T15)  [unwired: 9 in, 1 out]
          n233 = And(x=TRUE, y=w347) -> (x .and. y?=w348:bool)
          n234 = case shown="False" w348 {
            tunnel: w352 -> [w361 w363]
            frame False {
              n235 = call-poly <vilib>:"WPI_SolenoidSet.vi"("Value"=WPI_SolenoidValue."Forward", "SolenoidDevRef"=w361) -> ()  [unwired: 8 in, 2 out]
            }
            frame True {
              n236 = call-poly <vilib>:"WPI_SolenoidSet.vi"("Value"=WPI_SolenoidValue."Reverse", "SolenoidDevRef"=w363) -> ()  [unwired: 8 in, 2 out]
            }
          }
        }
        frame "Just fired", Default {
          # "When MicroSwitch is \nadded, Change this \nto read from that"
          n237 = local read "Timer for firing mech"() -> (w375:dbl)
          n238 = call <vilib>:"WPI_SolenoidRefNum Registry Get.vi"("refnum name"="Firing Pin Solenoid") -> ("error out"=w372:errorcluster, "SolenoidDevRef"=w371:T15)  [unwired: 9 in]
          n239 = Tick Count (ms)() -> (millisecond timer value=w374:u32)
          n240 = call-poly <vilib>:"WPI_SolenoidSet.vi"("error in (no error)"=w372, "Value"=WPI_SolenoidValue."Reverse", "SolenoidDevRef"=w371) -> ()  [unwired: 7 in, 2 out]
          n241 = Subtract(x=w374, y=w375) -> (x-y=w366:dbl)
          n242 = Greater Or Equal?(x=w366, y=3000) -> (x >= y?=w369:bool)
          n243 = And(x=TRUE, y=w369) -> (x .and. y?=w368:bool)
          n244 = case shown="True" w368 {
            frame False {
            }
            frame True {
              n245 = local write "Current Shooter Status"(T3."Pulling back" ("Current Shooter Status")) -> ()
            }
          }
        }
      }
    }
  }
  n246 = call <vilib>:"SD Read Boolean.vi"("Name"="Grabber Pistons Extended") -> ("Boolean"=w11:bool)  [unwired: 8 in, 2 out]
  n247 = case shown="\"Resetting\", Default" w46 {
    tunnel: ["Resetting" "Going Up" "Going Up Slow" "In Shooting Position" "Going Down" "Going Down Slow" "In Loading Position"] -> w45
    frame "Resetting", Default {
    }
    frame "Going Up" {
    }
    frame "Going Up Slow" {
    }
    frame "In Shooting Position" {
    }
    frame "Going Down" {
    }
    frame "Going Down Slow" {
    }
    frame "In Loading Position" {
    }
  }
  n248 = case shown="\"Retracting\", Default" w47 {
    tunnel: ["Retracting" "Firing" "Ready to fire" "Pulling back" "Just fired"] -> w44
    frame "Retracting", Default {
    }
    frame "Firing" {
    }
    frame "Ready to fire" {
    }
    frame "Pulling back" {
    }
    frame "Just fired" {
    }
  }
  n249 = call <vilib>:"WPI_EncoderGet.vi"("error in (no error)"=w50, "EncoderDevRef"=w51) -> ("Distance"=→"Waveform Chart 2":dbl)  [unwired: 4 in, 5 out]
  n250 = Equal?(x=w11, y=FALSE) -> (x = y?=w13:bool)
  n251 = Select(t=WPI_SolenoidValue."Forward" ("Value"), s=w13, f=WPI_SolenoidValue."Reverse") -> (s? t:f=w16:T6)
  n252 = call-poly <vilib>:"WPI_SolenoidSet.vi"("Value"=w16, "SolenoidDevRef"=w9) -> ()  [unwired: 8 in, 2 out]
  n253 = call <vilib>:"SD Write String.vi"("String"=w44, "Name"="Current Shooter Status") -> ()  [unwired: 8 in, 2 out]
  n254 = call <vilib>:"SD Write String.vi"("String"=w45, "Name"="Current Grabber Status") -> ()  [unwired: 8 in, 2 out]
  n255 = Multiply(x=w82, y=0.75) -> (x*y=w33:dbl)
  n256 = call <vilib>:"WPI_EncoderRefNum Registry Get.vi"("refnum name"="Left Drive Encoder") -> ("EncoderDevRef"=w5:T23)  [unwired: 9 in, 1 out]
  n257 = call <vilib>:"WPI_EncoderRefNum Registry Get.vi"("refnum name"="Right Drive Encoder") -> ("error out"=w7:errorcluster, "EncoderDevRef"=w6:T23)  [unwired: 9 in]
  n258 = call <vilib>:"WPI_DigitalInputRefNum Registry Get.vi"("refnum name"="Micro Switch 1") -> ("DigitalInputDevRef"=w30:T21)  [unwired: 9 in, 1 out]
  n259 = call <vilib>:"WPI_EncoderGet.vi"("error in (no error)"=w7, "EncoderDevRef"=w6) -> ("Distance"=→"Waveform Chart 4":dbl)  [unwired: 4 in, 5 out]
  n260 = call <vilib>:"WPI_EncoderGet.vi"("EncoderDevRef"=w5) -> ("Distance"=→"Waveform Chart 3":dbl)  [unwired: 5 in, 5 out]
  n261 = call <vilib>:"WPI_DigitalInputRefNum Registry Get.vi"("refnum name"="Bottom Limit Switch") -> ("DigitalInputDevRef"=w35:T21)  [unwired: 9 in, 1 out]
  n262 = call <vilib>:"WPI_DigitalInputRefNum Registry Get.vi"("refnum name"="Top Limit Switch") -> ("DigitalInputDevRef"=w27:T21)  [unwired: 9 in, 1 out]
  n263 = call <vilib>:"WPI_DigitalInputGetValue.vi"("DigitalInputDevRef"=w30) -> ("Value"=w31:bool)  [unwired: 8 in, 2 out]
  n264 = call <vilib>:"WPI_DigitalInputGetValue.vi"("DigitalInputDevRef"=w35) -> ("Value"=w22:bool)  [unwired: 8 in, 2 out]
  n265 = call <vilib>:"WPI_DigitalInputGetValue.vi"("DigitalInputDevRef"=w27) -> ("Value"=w8:bool)  [unwired: 8 in, 2 out]
  n266 = Not(x=w31) -> (.not. x?=w21:bool)
  n267 = Less?(x=w33, y=-0.01) -> (x < y?=w34:bool)
  n268 = And(x=w22, y=w21) -> (x .and. y?=w20:bool)
  n269 = And(x=w8, y=w21) -> (x .and. y?=w25:bool)
  n270 = Greater?(x=w33, y=0.01) -> (0:w26:bool)
  n271 = And(x=w20, y=w34) -> (x .and. y?=w23:bool)
  n272 = And(x=w26, y=w25) -> (x .and. y?=w24:bool)
  n273 = Or(x=w23, y=w24) -> (x .or. y?=w19:bool)
  n274 = case shown="True" w19 {
    tunnel: w33 -> [_ w392]
    frame False {
      n275 = call <vilib>:"WPI_MotorControlRefNum Registry Get.vi"("refnum name"="Fisher Price") -> ("MotorControlDevRef"=w390:T8)  [unwired: 9 in, 1 out]
      n276 = call <vilib>:"WPI_MotorControlSetOutput.vi"("Output"=0.0, "MotorControlDevRef"=w390) -> ()  [unwired: 7 in, 3 out]
    }
    frame True {
      n277 = call <vilib>:"WPI_MotorControlRefNum Registry Get.vi"("refnum name"="Fisher Price") -> ("MotorControlDevRef"=w394:T8)  [unwired: 9 in, 1 out]
      n278 = call <vilib>:"WPI_MotorControlSetOutput.vi"("Output"=w392, "MotorControlDevRef"=w394) -> ()  [unwired: 7 in, 3 out]
    }
  }
  n279 = call <vilib>:"WPI_JoystickRefNum Registry Get.vi"("refnum name"="Joystick 1") -> ("JoystickDevRef"=w148:T18)  [unwired: 1 in, 9 out]
  n280 = call <vilib>:"WPI_JoystickGet.vi"("JoystickDevRef"=w148) -> ("Buttons"=w146:T20, "Axes"=w143:T36)  [unwired: 1 in, 4 out]
  n281 = Unbundle By Name(w143) -> ("axis 1 (x)"=w112:dbl, "axis 2 (y)"=w110:dbl)  [unwired: 1 out]
  n282 = Cluster To Array(cluster=w143) -> (array=w142:dbl[])
  n283 = Cluster To Array(cluster=w146) -> (array=w145:bool[])
  n284 = Negate(x=w112) -> (-x=w111:dbl)
  n285 = Negate(x=w110) -> (-x=w109:dbl)
  n286 = call <vilib>:"WPI_RobotDriveRefNum Registry Get.vi"("refnum name"="Left and Right Motors") -> ("RobotDriveDevRef"=w150:T37)  [unwired: 1 in, 9 out]
  n287 = call <vilib>:"SD Write Numeric Array.vi"("Numeric Array"=w142, "Name"="Joystick 1/Axes") -> ()  [unwired: 8 in, 2 out]
  n288 = call <vilib>:"SD Write Boolean Array.vi"("Boolean Array"=w145, "Name"="Joystick 1/Buttons") -> ()  [unwired: 8 in, 2 out]
  n289 = call <vilib>:"WPI_RobotDriveArcadeDrive_Standard(NoSaturation).vi"("Y axis value"=w109, "X axis value"=w111, "RobotDriveDevRef"=w150) -> ("Motor Values"=w139:dbl[])  [unwired: 1 in, 7 out]
  n290 = call <vilib>:"SD Write Numeric Array.vi"("Numeric Array"=w139, "Name"="Robot Drive Motors") -> ()  [unwired: 8 in, 2 out]
